vi "Configure.vi"(8 "error in (no error)":errorcluster, 11 "Cascade512II in":refnum<class "DAQCascade512II.lvclass">) -> (0 "error out":errorcluster, 2 "cancelled?":bool, 3 "Cascade512II out":refnum<class "DAQCascade512II.lvclass">)   [LabVIEW 2012, in "DAQCascade512II.lvclass"]
doc: "The configure method configures the details for the RabbitMQ connection, the observers and the mapping script.\n\nIn the derived class, make a call to the parent for setting these parameters."
uses:
  DAQCascade512II.lvclass
  configuration cluster.ctl
  DAQCascade512II.lvclass/DAQCascade512II.ctl
  <vilib>/Distrio/Murmex/Murmex/Murmex.lvclass
panel:
  in  "configuration":T1={"Temperature"=0.0, "Acquire / Focus Flag  of trigger"=0, "Number of Images fo Initializer"=0, "Data Type"=0, "Timing Mode of trigger "=1, "Gain multiplication"=4095.0, "Fast ADC"=TRUE} {"Gain multiplication" min=0.0 max=4095.0 step=1.0 scale=0.0..4095.0; "Temperature" format="%.2f"}
  in  "button:ok":bool
  in  "button:cancle":bool
  in  "button:call parent":bool
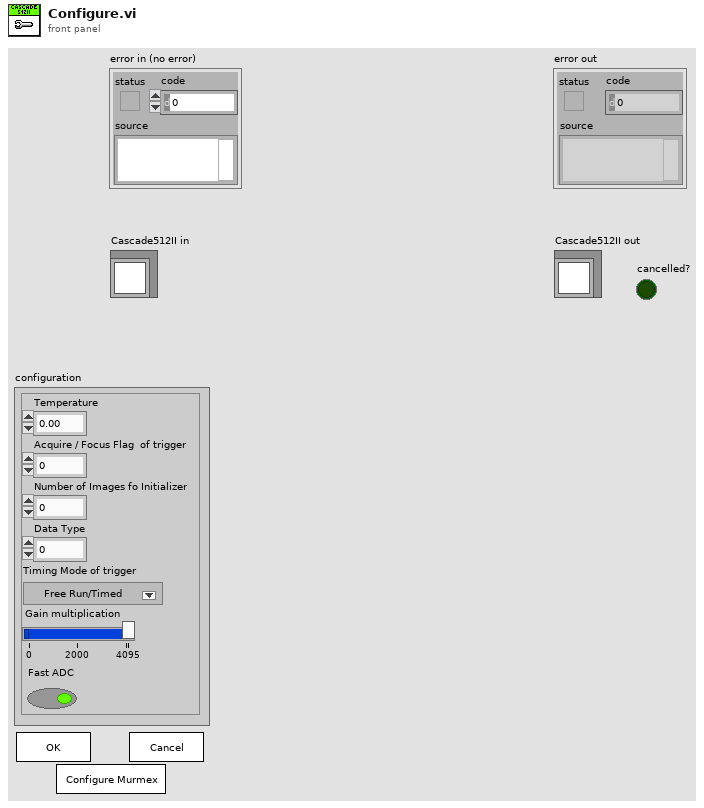
[diagram p1: front panel]
types:
  T1 = typedef "DAQCascade512II.lvclass/configuration cluster.ctl" = cluster{"Temperature":dbl, "Acquire / Focus Flag  of trigger":u32, "Number of Images fo Initializer":u32, "Data Type":u32, "Timing Mode of trigger ":u32, "Gain multiplication":dbl, "Fast ADC":bool}
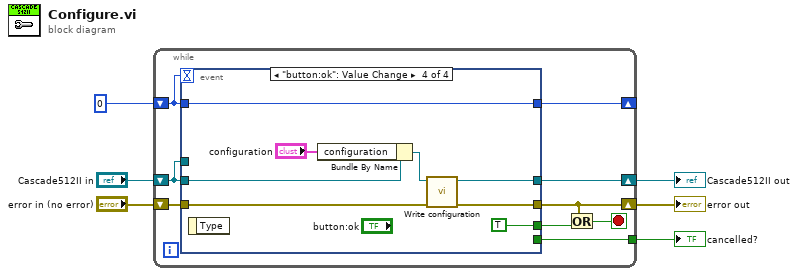
[diagram p0: block diagram]
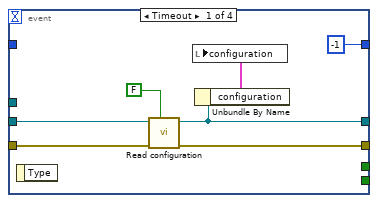
[diagram p2: hidden frame]
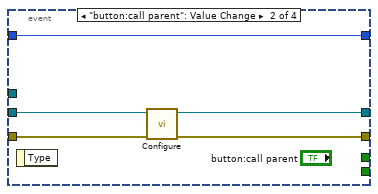
[diagram p3: hidden frame]
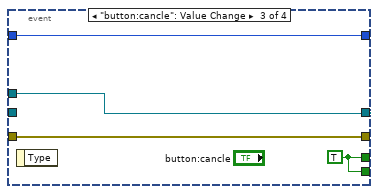
[diagram p4: hidden frame]
diagram:
  n1 = while {
    tunnel: [w13] -> w2
    shift-right: [w9] -> _
    shift-left: 0 -> [w8]
    shift-right: [w12] -> w6
    shift-left: "error in (no error)" -> [w14]
    shift-right: [w15] -> w1
    shift-left: "Cascade512II in" -> [w7]
    stop <- w10 stop-if-true
    n2 = event shown="[3] \"button:ok\": Value Change" {
      selector: _ -> [_ _ _ _]
      dyn-events: _ -> [_ _ _ _]
      timeout: w8 -> [_ _ _ _]
      tunnel: [w20 w25 w29 w37] -> w12
      tunnel: [w17 w24 w30 w35] -> w15
      tunnel: w14 -> [w21 w26 w29 w38]
      tunnel: w7 -> [w19 w27 _ w39]
      tunnel: w8 -> [_ w23 w31 w34]
      tunnel: [-1 w23 w31 w34] -> w9
      tunnel: [_ _ w28 _] -> w13
      tunnel: [_ _ w28 TRUE] -> w11
      tunnel: w7 -> [_ _ w30 _]
      event Timeout {
        n3 = event-data() -> ()  [unwired: 1 in, 1 out]
        n4 = call-dynamic "Read configuration.vi"("force loading?"=FALSE, "error in (no error)"=w21, "Cascade512II in"=w19) -> ("error out"=w20:errorcluster, "Cascade512II out"=w17:refnum<class "DAQCascade512II.lvclass">)  [unwired: 7 in]
        n5 = Unbundle By Name(w17) -> ("configuration"=w16:T1)
        n6 = local write "configuration"(w16) -> ()
      }
      event "button:call parent": Value Change {
        n7 = event-data() -> ()  [unwired: 1 in, 1 out]
        n8 = call-parent "Configure.vi"("error in (no error)"=w26, "Murmex in"=w27) -> ("error out"=w25:errorcluster, "Murmex out"=w24:refnum<class "DAQCascade512II.lvclass">)  [unwired: 7 in, 1 out]
      }
      event "button:cancle": Value Change {
        w28 = TRUE
        n9 = event-data() -> ()  [unwired: 1 in, 1 out]
      }
      event "button:ok": Value Change {
        n10 = event-data() -> ()  [unwired: 1 in, 1 out]
        n11 = Bundle By Name(cluster=w39, "configuration"="configuration") -> (w36:refnum<class "DAQCascade512II.lvclass">)
        n12 = call-dynamic "Write configuration.vi"("error in (no error)"=w38, "Cascade512II in"=w36) -> ("error out"=w37:errorcluster, "Cascade512II out"=w35:refnum<class "DAQCascade512II.lvclass">)  [unwired: 8 in]
      }
    }
    n13 = Or(x=w12, y=w11) -> (x .or. y?=w10:bool)
  }
  "error out" <- w6
  "Cascade512II out" <- w1
  "cancelled?" <- w2
